vi "Test Bit Conversion.vi"() -> ()   [LabVIEW 2013]
panel:
  out "16_bit_out":i16
  out "bits bool 8_15":bool[](array[boolean])
  out "bits bool 0_7":bool[](array[boolean])
  out "bits 0_7":u8
  in  "16bit":i16
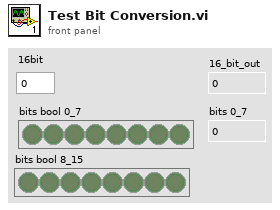
[diagram p1: front panel]
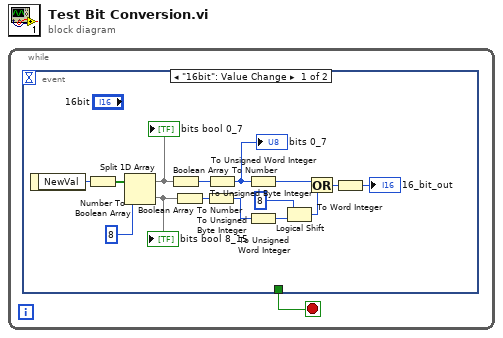
[diagram p0: block diagram]
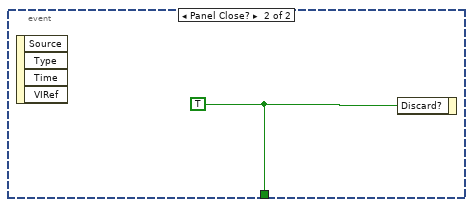
[diagram p2: hidden frame]
diagram:
  n1 = while {
    stop <- w1 stop-if-true
    n2 = event shown="[0] \"16bit\": Value Change" {
      selector: _ -> [_ _]
      dyn-events: _ -> [_ _]
      timeout: _ -> [_ _]
      tunnel: [_ w17] -> w1
      event "16bit": Value Change {
        n3 = event-data() -> ("NewVal"=w3:i16)  [unwired: 1 in]
        n4 = Number To Boolean Array(number=w3) -> (Boolean array=w4:bool[])
        n5 = Split 1D Array(array=w4, index=8) -> (first subarray=w6:bool[], second subarray=w7:bool[])
        "bits bool 0_7" <- w6
        "bits bool 8_15" <- w7
        n6 = Boolean Array To Number(Boolean array=w6) -> (number=w9:u32)
        n7 = Boolean Array To Number(Boolean array=w7) -> (number=w10:u32)
        n8 = To Unsigned Byte Integer(number=w10) -> (unsigned 8bit integer=w12:u8)
        n9 = To Unsigned Byte Integer(number=w9) -> (unsigned 8bit integer=w11:u8)
        "bits 0_7" <- w11
        n10 = To Unsigned Word Integer(number=w11) -> (unsigned 16bit integer=w14:u16)
        n11 = To Unsigned Word Integer(number=w12) -> (unsigned 16bit integer=w13:u16)
        n12 = Logical Shift(y=u16 8, x=w13) -> (x << y=w2:u16)
        n13 = Or(x=w14, y=w2) -> (x .or. y?=w15:u16)
        n14 = To Word Integer(number=w15) -> (16bit integer=→"16_bit_out":i16)
      }
      event Panel Close? {
        w17 = TRUE ("Discard?")
        n15 = event-data() -> ()  [unwired: 1 in, 4 out]
        n16 = event-data("Discard?"=w17) -> ()  [unwired: 1 in, 1 out]
      }
    }
  }
